vi "LSMcontroller_v59_PIzstage.vi"() -> ()   [LabVIEW 2015] (continued)
                    n3063 = property on="ROI" class="Bool (strict)"("Val(Sgnl)"=FALSE ("x/y scan")) -> ()  [unwired: 2 in, 2 out]
                  }
                }
              }
            }
          }
          event "Xdattype": Value Change {
            n3064 = event-data() -> ()  [unwired: 1 in, 1 out]
            n3065 = case shown="True" "Xdattype" {
              frame False {
              }
              frame True {
                n3066 = stacked-sequence {
                  frame #0 {
                    n3067 = Current VI's Path() -> (path=w6265:path)
                    n3068 = Strip Path(path=w6265) -> (stripped path=w6266:path)  [unwired: 1 out]
                    n3069 = Build Path(base path=w6266, name or relative path="subVIs\\Misc\\Changedataconfig.vi") -> (appended path=w6264:path)
                    n3070 = call <vilib>:"Set Busy.vi"() -> ("error out"=w6262:errorcluster)  [unwired: 10 in, 1 out]
                    n3071 = Open VI Reference(type specifier VI Refnum (for type only)=refnum<vi> refnum, vi path=w6264, error in (no error)=w6262) -> (vi reference=w6257:refnum<vi>, error out=w6259:errorcluster)  [unwired: 3 in]
                    n3072 = call-by-ref "?"(reference=w6257, error in=w6259) -> (reference out=w6261:refnum<vi>, error out=w6260:errorcluster)  [unwired: 12 in]
                    n3073 = Close Reference(reference=w6261, error in (no error)=w6260) -> (error out=w6256:errorcluster)
                    "status" <- w6256
                    n3074 = call <vilib>:"Unset Busy.vi"("error in (no error)"=w6256) -> ()  [unwired: 10 in, 1 out]
                  }
                  frame #1 {
                    n3075 = property on="Xdattype" class="Bool (strict)"("Val(Sgnl)"=FALSE ("x/y scan")) -> ()  [unwired: 2 in, 2 out]
                  }
                }
              }
            }
          }
          event "XautoOD": Value Change {
            n3076 = event-data() -> ()  [unwired: 1 in, 1 out]
            n3077 = case shown="True" "XautoOD" {
              frame False {
              }
              frame True {
                n3078 = stacked-sequence {
                  frame #0 {
                    n3079 = Current VI's Path() -> (path=w6278:path)
                    n3080 = Strip Path(path=w6278) -> (stripped path=w6279:path)  [unwired: 1 out]
                    n3081 = Build Path(base path=w6279, name or relative path="subVIs\\Misc\\ChangeautoODs.vi") -> (appended path=w6277:path)
                    n3082 = call <vilib>:"Set Busy.vi"() -> ("error out"=w6275:errorcluster)  [unwired: 10 in, 1 out]
                    n3083 = Open VI Reference(type specifier VI Refnum (for type only)=refnum<vi> refnum, vi path=w6277, error in (no error)=w6275) -> (vi reference=w6270:refnum<vi>, error out=w6272:errorcluster)  [unwired: 3 in]
                    n3084 = call-by-ref "?"(reference=w6270, error in=w6272) -> (reference out=w6274:refnum<vi>, error out=w6273:errorcluster)  [unwired: 12 in]
                    n3085 = Close Reference(reference=w6274, error in (no error)=w6273) -> (error out=w6269:errorcluster)
                    "status 2" <- w6269
                    n3086 = call <vilib>:"Unset Busy.vi"("error in (no error)"=w6269) -> ()  [unwired: 10 in, 1 out]
                  }
                  frame #1 {
                    n3087 = property on="XautoOD" class="Bool (strict)"("Val(Sgnl)"=FALSE ("x/y scan")) -> ()  [unwired: 2 in, 2 out]
                  }
                }
              }
            }
          }
          event "SetMan": Value Change {
            n3088 = event-data() -> ()  [unwired: 1 in, 1 out]
            n3089 = case shown="True" "SetMan" {
              frame False {
              }
              frame True {
                n3090 = stacked-sequence {
                  frame #0 {
                    w6282 = u16 0 items=["Rectangle", "Circle", "Freeform Boundary", "Freeform Interior"] ("ROI Type")
                    n3091 = local write "ROI Type"(w6282) -> ()
                    n3092 = local read "Square pixels"() -> (w6288:bool)
                    n3093 = case shown="True" w6288 {
                      frame False {
                        n3094 = local read "square matrix"() -> (w6289:bool)
                        n3095 = case shown="False" w6289 {
                          frame False {
                            "ypixels ref" <- "ypixels"
                            "xpixels ref" <- "xpixels"
                          }
                          frame True {
                            n3096 = local read "xpixels"() -> (w6294:i32)
                            n3097 = local read "ypixels"() -> (w6293:i32)
                            n3098 = Max & Min(x=w6294, y=w6293) -> (max(x,y)=w6292:i32)  [unwired: 1 out]
                            n3099 = local write "xpixels ref"(w6292) -> ()
                            n3100 = local write "ypixels ref"(w6292) -> ()
                          }
                        }
                      }
                      frame True {
                        n3101 = local read "square matrix"() -> (w6295:bool)
                        n3102 = case shown="False" w6295 {
                          frame False {
                            n3103 = local read "Vxmax"() -> (w6309:dbl)
                            n3104 = local read "Vx-min"() -> (w6308:dbl)
                            n3105 = local read "Vy-max"() -> (w6304:dbl)
                            n3106 = local read "Vy-min"() -> (w6305:dbl)
                            n3107 = Subtract(x=w6304, y=w6305) -> (x-y=w6306:dbl)
                            n3108 = Subtract(x=w6309, y=w6308) -> (x-y=w6307:dbl)
                            n3109 = Absolute Value(x=w6306) -> (abs(x)=w6297:dbl)
                            n3110 = Absolute Value(x=w6307) -> (abs(x)=w6298:dbl)
                            n3111 = Divide(x=w6298, y=w6297) -> (x/y=w6303:dbl)
                            n3112 = Greater Or Equal?(x=w6298, y=w6297) -> (x >= y?=w6296:bool)
                            n3113 = local read "xpixels"() -> (w6302:i32)
                            n3114 = local read "ypixels"() -> (w6299:i32)
                            n3115 = case shown="False" w6296 {
                              tunnel: w6303 -> [w6314 w6317]
                              tunnel: w6302 -> [w6311 _]
                              tunnel: [w6311 w6316] -> w6301
                              tunnel: [w6310 w6315] -> w6300
                              tunnel: w6299 -> [_ w6315]
                              frame False {
                                n3116 = To Double Precision Float(number=w6311) -> (double precision float=w6313:dbl)
                                n3117 = Divide(x=w6313, y=w6314) -> (x/y=w6312:dbl)
                                n3118 = To Long Integer(number=w6312) -> (32bit integer=w6310:i32)
                              }
                              frame True {
                                n3119 = To Double Precision Float(number=w6315) -> (double precision float=w6319:dbl)
                                n3120 = Multiply(x=w6319, y=w6317) -> (x*y=w6318:dbl)
                                n3121 = To Long Integer(number=w6318) -> (32bit integer=w6316:i32)
                              }
                            }
                            n3122 = local write "ypixels ref"(w6300) -> ()
                            n3123 = local write "xpixels ref"(w6301) -> ()
                          }
                          frame True {
                          }
                        }
                      }
                    }
                    "Vx-max ref" <- "Vxmax"
                    "Vx-min ref" <- "Vx-min"
                    "Vy-max ref" <- "Vy-max"
                    "Vy-min ref" <- "Vy-min"
                    "Angle ref" <- "Angle"
                  }
                  frame #1 {
                    n3124 = property on="SetMan" class="Bool (strict)"("Val(Sgnl)"=FALSE ("Value (Signaling)")) -> ()  [unwired: 2 in, 2 out]
                  }
                }
              }
            }
          }
          event "SetMan 2": Value Change {
            n3125 = event-data() -> ()  [unwired: 1 in, 1 out]
            n3126 = case shown="True" "SetMan 2" {
              frame False {
              }
              frame True {
                n3127 = stacked-sequence {
                  frame #0 {
                    n3128 = local write "Vx-ref"("Vx") -> ()
                    n3129 = local write "Vy-ref"("Vy") -> ()
                  }
                  frame #1 {
                    n3130 = property on="SetMan 2" class="Bool (strict)"("Val(Sgnl)"=FALSE ("Value (Signaling)")) -> ()  [unwired: 2 in, 2 out]
                  }
                }
              }
            }
          }
          event "Reset Coords": Value Change {
            n3131 = event-data() -> ("NewVal"=w6325:bool)  [unwired: 1 in, 5 out]
            n3132 = case shown="True" w6325 {
              frame False {
              }
              frame True {
                n3133 = stacked-sequence {
                  frame #0 {
                    n3134 = local write "xpixels"(256 ("xpixels")) -> ()
                    n3135 = local write "ypixels"(256 ("ypixels")) -> ()
                    n3136 = local write "Vxmax"(9.0 ("Vx-max")) -> ()
                    n3137 = local write "Vx-min"(-9.0 ("Vx-min")) -> ()
                    n3138 = local write "Vy-max"(9.0 ("Vy-max")) -> ()
                    n3139 = local write "Vy-min"(-9.0 ("Vy-min")) -> ()
                    n3140 = local write "Angle"(0.0 ("Angle")) -> ()
                  }
                  frame #1 {
                    n3141 = property on="Reset Coords" class="Bool (strict)"("Value"=FALSE ("TROI")) -> ()  [unwired: 2 in, 2 out]
                  }
                }
              }
            }
          }
          event "TROI": Value Change {
            n3142 = event-data() -> ()  [unwired: 1 in, 1 out]
            n3143 = case shown="True" "TROI" {
              frame False {
              }
              frame True {
                n3144 = stacked-sequence {
                  frame #0 {
                    n3145 = local read "Vy-min ref"() -> (w6339:dbl)
                    n3146 = local read "Vy-max ref"() -> (w6338:dbl)
                    n3147 = local read "Vx-max ref"() -> (w6336:dbl)
                    n3148 = local read "Vx-min ref"() -> (w6337:dbl)
                    n3149 = local read "ypixels ref"() -> (w6341:i32)
                    n3150 = local read "xpixels ref"() -> (w6340:i32)
                    n3151 = local read "Angle ref"() -> (w6335:dbl)
                    n3152 = local write "Angle"(w6335) -> ()
                    n3153 = local write "xpixels"(w6340) -> ()
                    n3154 = local write "Vy-min"(w6339) -> ()
                    n3155 = local write "Vy-max"(w6338) -> ()
                    n3156 = local write "Vx-min"(w6337) -> ()
                    n3157 = local write "ypixels"(w6341) -> ()
                    n3158 = local write "Vxmax"(w6336) -> ()
                  }
                  frame #1 {
                    n3159 = property on="TROI" class="Bool (strict)"("Value"=FALSE ("TROI")) -> ()  [unwired: 2 in, 2 out]
                  }
                }
              }
            }
          }
          event "TROI 2": Value Change {
            n3160 = event-data() -> ()  [unwired: 1 in, 1 out]
            n3161 = case shown="True" "TROI 2" {
              frame False {
              }
              frame True {
                n3162 = stacked-sequence {
                  frame #0 {
                    n3163 = local read "Vx-ref"() -> (w6344:dbl)
                    n3164 = local read "Vy-ref"() -> (w6345:dbl)
                    n3165 = local write "Vx"(w6344) -> ()
                    n3166 = local write "Vy"(w6345) -> ()
                  }
                  frame #1 {
                    n3167 = property on="TROI 2" class="Bool (strict)"("Value"=FALSE ("TROI")) -> ()  [unwired: 2 in, 2 out]
                  }
                }
              }
            }
          }
          event "Square pixels": Value Change {
            n3168 = event-data() -> ()  [unwired: 1 in, 1 out]
            n3169 = case shown="True" "Square pixels" {
              frame False {
              }
              frame True {
                n3170 = property on="square matrix" class="Bool (strict)"("Value"=FALSE ("square matrix")) -> ()  [unwired: 2 in, 2 out]
                n3171 = property on="Square pixels" class="Bool (strict)"("Value"=TRUE ("square matrix")) -> ()  [unwired: 2 in, 2 out]
              }
            }
          }
          event "square matrix": Value Change {
            n3172 = event-data() -> ()  [unwired: 1 in, 1 out]
            n3173 = case shown="True" "square matrix" {
              frame False {
              }
              frame True {
                n3174 = property on="square matrix" class="Bool (strict)"("Value"=TRUE ("square matrix")) -> ()  [unwired: 2 in, 2 out]
                n3175 = property on="Square pixels" class="Bool (strict)"("Value"=FALSE ("square matrix")) -> ()  [unwired: 2 in, 2 out]
              }
            }
          }
          event "up", "downright", "down", "downleft", "right", "left", "upright", "upleft": Value Change {
            n3176 = event-data() -> ()  [unwired: 1 in, 6 out]
            n3177 = local read "downright"() -> (w6358:bool)
            n3178 = local read "downleft"() -> (w6360:bool)
            n3179 = local read "upright"() -> (w6356:bool)
            n3180 = local read "upleft"() -> (w6354:bool)
            n3181 = local read "down"() -> (w6359:bool)
            n3182 = local read "right"() -> (w6357:bool)
            n3183 = local read "left"() -> (w6361:bool)
            n3184 = local read "up"() -> (w6355:bool)
            n3185 = Compound Arithmetic op=OR(w6354, w6355, w6356, w6357, w6358, w6359, w6360, w6361) -> (w6353:bool)
            n3186 = case shown="True" w6353 {
              frame False {
              }
              frame True {
                n3187 = stacked-sequence {
                  frame #0 {
                    n3188 = local read "downright"() -> (w6363:bool)
                    n3189 = local read "downleft"() -> (w6365:bool)
                    n3190 = local read "BigSmall"() -> (w6362:bool)
                    n3191 = local read "upright"() -> (w6367:bool)
                    n3192 = local read "upleft"() -> (w6370:bool)
                    n3193 = local read "down"() -> (w6366:bool)
                    n3194 = local read "right"() -> (w6368:bool)
                    n3195 = local read "left"() -> (w6364:bool)
                    n3196 = local read "up"() -> (w6369:bool)
                    n3197 = call "movestageparams.vi"("command"="get") -> ("Params out"=w6373:T21)  [unwired: 1 in]
                    n3198 = Bundle By Name(cluster=w6373, "upleft"=w6370, "up"=w6369, "upright"=w6367, "right"=w6368, "downright"=w6363, "down"=w6366, "downleft"=w6365, "left"=w6364, "Bigsmall"=w6362) -> (w6374:T21)
                    n3199 = call "movestageparams.vi"("Params in"=w6374, "command"="set") -> ()  [unwired: 1 out]
                  }
                  frame #1 {
                    n3200 = disable-structure shown="Disabled" {
                      frame Disabled {
                        n3201 = call "configuration.vi"("command"="get") -> ("config out"=w6377:T12)  [unwired: 2 in, 1 out]
                        n3202 = in-place {
                          n3203 = in-place-cluster #45(w6377) -> ()  [unwired: 2 out]
                          n3204 = in-place-cluster #45("StageL"="StageL", "StageS"="StageS") -> (w6375:T12)
                        }
                        n3205 = call "configuration.vi"("config in"=w6375, "command"="set") -> ()  [unwired: 1 in, 2 out]
                      }
                      frame Enabled {
                      }
                    }
                  }
                  frame #2 {
                    n3206 = call "movestage.vi"() -> ()  [unwired: 12 in]
                  }
                  frame #3 {
                    w6381 = FALSE ("OK Button")
                    w6382 = FALSE ("OK Button")
                    n3207 = property on="down" class="Bool (strict)"("Value"=w6382) -> ()  [unwired: 2 in, 2 out]
                    n3208 = property on="up" class="Bool (strict)"("Value"=w6382) -> ()  [unwired: 2 in, 2 out]
                    n3209 = property on="right" class="Bool (strict)"("Value"=w6382) -> ()  [unwired: 2 in, 2 out]
                    n3210 = property on="left" class="Bool (strict)"("Value"=w6382) -> ()  [unwired: 2 in, 2 out]
                    n3211 = property on="upright" class="Bool (strict)"("Value"=w6381) -> ()  [unwired: 2 in, 2 out]
                    n3212 = property on="downleft" class="Bool (strict)"("Value"=w6381) -> ()  [unwired: 2 in, 2 out]
                    n3213 = property on="downright" class="Bool (strict)"("Value"=w6381) -> ()  [unwired: 2 in, 2 out]
                    n3214 = property on="upleft" class="Bool (strict)"("Value"=w6381) -> ()  [unwired: 2 in, 2 out]
                  }
                }
              }
            }
          }
          event "finite samples": Value Change {
            n3215 = event-data() -> ("NewVal"=w6383:bool)  [unwired: 1 in]
            n3216 = flat-sequence {
              tunnel: w6383 -> [w6384]
              frame #0 {
                n3217 = case shown="True" w6384 {
                  frame False {
                    w6385 = FALSE ("wavdet")
                    n3218 = property on="continuous" class="Bool (strict)"("Value"=TRUE ("continuous for display")) -> ()  [unwired: 2 in, 2 out]
                    n3219 = property on="wavdet" class="Bool (strict)"("Value"=w6385) -> ()  [unwired: 2 in, 2 out]
                    n3220 = property on="save\ndata" class="Bool (strict)"("Value"=w6385) -> ()  [unwired: 2 in, 2 out]
                    n3221 = property on="# of frames" class="DigNum (strict)"("DisabledEnum"=T7."Disabled and Grayed Out" ("Disabled")) -> ()  [unwired: 2 in, 2 out]
                    n3222 = property on="save\ndata" class="Bool (strict)"("DisabledEnum"=T7."Disabled and Grayed Out" ("Disabled")) -> ()  [unwired: 2 in, 2 out]
                    "Save tab" <- enum32{"withsave", "withoutsave"}."withsave" ("Save tab")
                  }
                  frame True {
                    w6392 = FALSE ("continuous for display")
                    n3223 = property on="continuous" class="Bool (strict)"("Value"=w6392) -> ()  [unwired: 2 in, 2 out]
                    n3224 = property on="wavdet" class="Bool (strict)"("Value"=w6392) -> ()  [unwired: 2 in, 2 out]
                    n3225 = local write "Save tab"(enum32{"withsave", "withoutsave"}."withsave" ("Save tab")) -> ()
                    n3226 = property on="save\ndata" class="Bool (strict)"("DisabledEnum"=T7."Enabled" ("Disabled")) -> ()  [unwired: 2 in, 2 out]
                    n3227 = property on="save\ndata" class="Bool (strict)"("Value"=TRUE ("save\ndata")) -> ()  [unwired: 2 in, 2 out]
                    n3228 = property on="# of frames" class="DigNum (strict)"("DisabledEnum"=T7."Enabled" ("Disabled")) -> ()  [unwired: 2 in, 2 out]
                  }
                }
              }
              frame #1 {
                n3229 = local read "finite samples"() -> (w6401:bool)
                n3230 = local read "continuous"() -> (w6400:bool)
                n3231 = local read "wavdet"() -> (w6399:bool)
                n3232 = call "2pparameters.vi"("command"="get") -> ("params out"=w6395:T11)  [unwired: 1 in]
                n3233 = Bundle By Name(cluster=w6395, "finite"=w6401, "cont"=w6400, "wavdet"=w6399) -> (w6398:T11)
                n3234 = call "2pparameters.vi"("Params in"=w6398, "command"="set") -> ()  [unwired: 1 out]
              }
            }
          }
          event "continuous": Value Change {
            n3235 = event-data() -> ("NewVal"=w6402:bool)  [unwired: 1 in]
            n3236 = flat-sequence {
              tunnel: w6402 -> [w6403]
              frame #0 {
                n3237 = case shown="True" w6403 {
                  frame False {
                    n3238 = property on="finite samples" class="Bool (strict)"("Value"=TRUE ("finite samples for recording")) -> ()  [unwired: 2 in, 2 out]
                    n3239 = property on="save\ndata" class="Bool (strict)"("Value"=TRUE ("save\ndata")) -> ()  [unwired: 2 in, 2 out]
                    n3240 = property on="wavdet" class="Bool (strict)"("Value"=FALSE ("wavdet")) -> ()  [unwired: 2 in, 2 out]
                    n3241 = local write "Save tab"(enum32{"withsave", "withoutsave"}."withsave" ("Save tab")) -> ()
                    n3242 = property on="# of frames" class="DigNum (strict)"("DisabledEnum"=T7."Enabled" ("Disabled")) -> ()  [unwired: 2 in, 2 out]
                    n3243 = property on="save\ndata" class="Bool (strict)"("DisabledEnum"=T7."Enabled" ("Disabled")) -> ()  [unwired: 2 in, 2 out]
                  }
                  frame True {
                    w6410 = FALSE ("finite samples for recording")
                    n3244 = property on="finite samples" class="Bool (strict)"("Value"=w6410) -> ()  [unwired: 2 in, 2 out]
                    n3245 = property on="wavdet" class="Bool (strict)"("Value"=w6410) -> ()  [unwired: 2 in, 2 out]
                    n3246 = property on="save\ndata" class="Bool (strict)"("Value"=w6410) -> ()  [unwired: 2 in, 2 out]
                    n3247 = local write "Save tab"(enum32{"withsave", "withoutsave"}."withsave" ("Save tab")) -> ()
                    n3248 = property on="# of frames" class="DigNum (strict)"("DisabledEnum"=T7."Disabled and Grayed Out" ("Disabled")) -> ()  [unwired: 2 in, 2 out]
                    n3249 = property on="save\ndata" class="Bool (strict)"("DisabledEnum"=T7."Disabled and Grayed Out" ("Disabled")) -> ()  [unwired: 2 in, 2 out]
                  }
                }
              }
              frame #1 {
                n3250 = local read "finite samples"() -> (w6420:bool)
                n3251 = local read "continuous"() -> (w6419:bool)
                n3252 = local read "wavdet"() -> (w6418:bool)
                n3253 = call "2pparameters.vi"("command"="get") -> ("params out"=w6414:T11)  [unwired: 1 in]
                n3254 = Bundle By Name(cluster=w6414, "finite"=w6420, "cont"=w6419, "wavdet"=w6418) -> (w6417:T11)
                n3255 = call "2pparameters.vi"("Params in"=w6417, "command"="set") -> ()  [unwired: 1 out]
              }
            }
          }
          event "wavdet": Value Change {
            n3256 = event-data() -> ("NewVal"=w6421:bool)  [unwired: 1 in]
            n3257 = flat-sequence {
              tunnel: w6421 -> [w6422]
              frame #0 {
                n3258 = case shown="False" w6422 {
                  frame False {
                    n3259 = property on="finite samples" class="Bool (strict)"("Value"=TRUE ("finite samples for recording")) -> ()  [unwired: 2 in, 2 out]
                    n3260 = property on="continuous" class="Bool (strict)"("Value"=FALSE ("continuous")) -> ()  [unwired: 2 in, 2 out]
                    n3261 = local write "Save tab"(enum32{"withsave", "withoutsave"}."withsave" ("Save tab")) -> ()
                    n3262 = property on="save\ndata" class="Bool (strict)"("DisabledEnum"=T7."Enabled" ("Disabled")) -> ()  [unwired: 2 in, 2 out]
                    n3263 = property on="# of frames" class="DigNum (strict)"("DisabledEnum"=T7."Enabled" ("Disabled")) -> ()  [unwired: 2 in, 2 out]
                    n3264 = property on="save\ndata" class="Bool (strict)"("Value"=TRUE ("save\ndata")) -> ()  [unwired: 2 in, 2 out]
                  }
                  frame True {
                    w6431 = FALSE ("finite samples for recording")
                    n3265 = property on="finite samples" class="Bool (strict)"("Value"=w6431) -> ()  [unwired: 2 in, 2 out]
                    n3266 = property on="continuous" class="Bool (strict)"("Value"=w6431) -> ()  [unwired: 2 in, 2 out]
                    n3267 = property on="save\ndata" class="Bool (strict)"("DisabledEnum"=T7."Enabled" ("Disabled")) -> ()  [unwired: 2 in, 2 out]
                    n3268 = local write "Save tab"(enum32{"withsave", "withoutsave"}."withsave" ("Save tab")) -> ()
                    n3269 = property on="# of frames" class="DigNum (strict)"("DisabledEnum"=T7."Disabled" ("Disabled")) -> ()  [unwired: 2 in, 2 out]
                    n3270 = property on="save\ndata" class="Bool (strict)"("Value"=TRUE ("save\ndata")) -> ()  [unwired: 2 in, 2 out]
                  }
                }
              }
              frame #1 {
                n3271 = local read "finite samples"() -> (w6434:bool)
                n3272 = local read "continuous"() -> (w6435:bool)
                n3273 = local read "wavdet"() -> (w6436:bool)
                n3274 = call "2pparameters.vi"("command"="get") -> ("params out"=w6440:T11)  [unwired: 1 in]
                n3275 = Bundle By Name(cluster=w6440, "finite"=w6434, "cont"=w6435, "wavdet"=w6436) -> (w6437:T11)
                n3276 = call "2pparameters.vi"("Params in"=w6437, "command"="set") -> ()  [unwired: 1 out]
              }
            }
          }
          event "cursors": Value Change {
            n3277 = event-data() -> ()  [unwired: 1 in, 5 out]
            n3278 = case shown="True" "cursors" {
              frame False {
                n3279 = property on="img_CH1" class="IntGraph (strict)"("Active Cursor"=u32 0, "Cursor.Cursor Style"=u8 0 ("Cursor Style"), "Cursor.Cursor Point Style"=u8 0 ("Cursor Point Style")) -> ("Cursor.Cursor Position:Cursor X"=w6445:dbl, "Cursor.Cursor Position:Cursor Y"=w6446:dbl)  [unwired: 2 in, 2 out]
                n3280 = property on="img_CH2" class="IntGraph (strict)"("Active Cursor"=u32 0, "Cursor.Cursor Style"=u8 0 ("Cursor Style"), "Cursor.Cursor Point Style"=u8 0 ("Cursor Point Style")) -> ()  [unwired: 2 in, 2 out]
                n3281 = local write "cursor x [pixel]"(w6445) -> ()
                n3282 = local write "cursor y [pixel]"(w6446) -> ()
              }
              frame True {
                n3283 = stacked-sequence {
                  frame #0 {
                    n3284 = call "2pparameters.vi"("command"="get") -> ("params out"=w6461:T11)  [unwired: 1 in]
                    n3285 = Unbundle By Name(w6461) -> ("Xpixels Img"=w6462:i32, "Ypixels Img"=w6459:i32)
                    n3286 = To Double Precision Float(number=w6459) -> (double precision float=w6453:dbl)
                    n3287 = To Double Precision Float(number=w6462) -> (double precision float=w6458:dbl)
                    n3288 = Divide(x=w6453, y=2.0) -> (x/y=w6454:dbl)
                    n3289 = Divide(x=w6458, y=2.0) -> (x/y=w6456:dbl)
                    n3290 = Round To Nearest(number=w6454) -> (nearest integer value=w6452:dbl)
                    n3291 = Round To Nearest(number=w6456) -> (nearest integer value=w6455:dbl)
                    n3292 = property on="img_CH1" class="IntGraph (strict)"("Active Cursor"=u32 0, "Cursor.Cursor Style"=u8 8 ("Cursor Style"), "Cursor.Cursor Point Style"=u8 5 ("Cursor Point Style"), "Cursor.Cursor Position:Cursor X"=w6455, "Cursor.Cursor Position:Cursor Y"=w6452, "Cursor.Visible"=TRUE) -> ()  [unwired: 2 in, 2 out]
                  }
                  frame #1 {
                    n3293 = call "2pparameters.vi"("command"="get") -> ("params out"=w6481:T11)  [unwired: 1 in]
                    n3294 = call "2pparameters.vi"("command"="get") -> ("params out"=w6479:T11)  [unwired: 1 in]
                    n3295 = property on="img_CH1" class="IntGraph (strict)"("Active Cursor"=u32 0, "Cursor.Cursor Style"=u8 8 ("Cursor Style"), "Cursor.Cursor Point Style"=u8 5 ("Cursor Point Style")) -> ("Cursor.Cursor Position:Cursor X"=w6474:dbl, "Cursor.Cursor Position:Cursor Y"=w6473:dbl, "Cursor.Cursor Index"=w6496:i32, "Cursor.Cursor Plot"=w6495:i32, "Cursor.Visible"=w6466:bool)  [unwired: 2 in, 2 out]
                    "cursor x [pixel]" <- w6474
                    "cursor y [pixel]" <- w6473
                    n3296 = Unbundle By Name(w6481) -> ("Vy-max Img"=w6483:dbl, "Vy-min Img"=w6470:dbl, "Ypixels Img"=w6485:i32)
                    n3297 = Unbundle By Name(w6479) -> ("VX-max Img"=w6480:dbl, "Vx-min Img"=w6468:dbl, "Xpixels Img"=w6484:i32)
                    n3298 = Subtract(x=w6483, y=w6470) -> (x-y=w6488:dbl)
                    n3299 = Subtract(x=w6480, y=w6468) -> (x-y=w6486:dbl)
                    n3300 = local read "img_CH2"() -> (w6492:sgl[][])
                    n3301 = To Double Precision Float(number=w6484) -> (double precision float=w6487:dbl)
                    n3302 = local read "img_CH1"() -> (w6493:sgl[][])
                    n3303 = To Double Precision Float(number=w6485) -> (double precision float=w6489:dbl)
                    n3304 = Index Array(array=w6493, index (row)=w6496, index (col)=w6495) -> (element=→"value CH 1":sgl)
                    n3305 = Index Array(array=w6492, index (row)=w6496, index (col)=w6495) -> (element=→"value CH 2":sgl)
                    n3306 = Divide(x=w6486, y=w6487) -> (x/y=w6490:dbl)
                    n3307 = Divide(x=w6488, y=w6489) -> (x/y=w6491:dbl)
                    n3308 = Multiply(x=w6474, y=w6490) -> (x*y=w6469:dbl)
                    n3309 = Multiply(x=w6473, y=w6491) -> (x*y=w6472:dbl)
                    n3310 = property on="img_CH2" class="IntGraph (strict)"("Active Cursor"=u32 0, "Cursor.Cursor Style"=u8 8 ("Cursor Style"), "Cursor.Cursor Point Style"=u8 5 ("Cursor Point Style"), "Cursor.Cursor Position:Cursor X"=w6474, "Cursor.Cursor Position:Cursor Y"=w6473, "Cursor.Visible"=w6466) -> ()  [unwired: 2 in, 2 out]
                    n3311 = Add(x=w6469, y=w6468) -> (x+y=w6467:dbl)
                    n3312 = Add(x=w6472, y=w6470) -> (x+y=w6471:dbl)
                    n3313 = local write "Vx-ref"(w6467) -> ()
                    n3314 = local write "Vy-ref"(w6471) -> ()
                  }
                }
              }
            }
          }
          event "img_CH1": Cursor Move {
            n3315 = event-data() -> ("CursIdx"=w6501:i32)  [unwired: 1 in]
            n3316 = Equal To 0?(x=w6501) -> (x = 0?=w6502:bool)
            n3317 = case shown="True" w6502 {
              frame False {
              }
              frame True {
                n3318 = call "2pparameters.vi"("command"="get") -> ("params out"=w6522:T11)  [unwired: 1 in]
                n3319 = call "2pparameters.vi"("command"="get") -> ("params out"=w6524:T11)  [unwired: 1 in]
                n3320 = property on="img_CH1" class="IntGraph (strict)"("Active Cursor"=u32 0, "Cursor.Cursor Style"=u8 8 ("Cursor Style"), "Cursor.Cursor Point Style"=u8 5 ("Cursor Point Style")) -> ("Cursor.Cursor Position:Cursor X"=w6511:dbl, "Cursor.Cursor Position:Cursor Y"=w6510:dbl, "Cursor.Cursor Plot"=w6530:i32, "Cursor.Cursor Index"=w6529:i32, "Cursor.Visible"=w6503:bool)  [unwired: 2 in, 2 out]
                n3321 = Unbundle By Name(w6522) -> ("Vy-max Img"=w6520:dbl, "Vy-min Img"=w6509:dbl, "Ypixels Img"=w6518:i32)
                n3322 = Unbundle By Name(w6524) -> ("VX-max Img"=w6523:dbl, "Vx-min Img"=w6504:dbl, "Xpixels Img"=w6519:i32)
                n3323 = Subtract(x=w6520, y=w6509) -> (x-y=w6515:dbl)
                n3324 = Subtract(x=w6523, y=w6504) -> (x-y=w6517:dbl)
                n3325 = local write "cursor x [pixel]"(w6511) -> ()
                n3326 = local write "cursor y [pixel]"(w6510) -> ()
                n3327 = To Double Precision Float(number=w6519) -> (double precision float=w6516:dbl)
                n3328 = To Double Precision Float(number=w6518) -> (double precision float=w6514:dbl)
                n3329 = local read "img_CH2"() -> (w6531:sgl[][])
                n3330 = local read "img_CH1"() -> (w6534:sgl[][])
                n3331 = Index Array(array=w6531, index (row)=w6530, index (col)=w6529) -> (element=w6532:sgl)
                n3332 = Index Array(array=w6534, index (row)=w6530, index (col)=w6529) -> (element=w6533:sgl)
                n3333 = Divide(x=w6517, y=w6516) -> (x/y=w6513:dbl)
                n3334 = Divide(x=w6515, y=w6514) -> (x/y=w6512:dbl)
                n3335 = local write "value CH 2"(w6532) -> ()
                n3336 = Multiply(x=w6511, y=w6513) -> (x*y=w6506:dbl)
                n3337 = local write "value CH 1"(w6533) -> ()
                n3338 = Multiply(x=w6510, y=w6512) -> (x*y=w6508:dbl)
                n3339 = Add(x=w6506, y=w6504) -> (x+y=w6505:dbl)
                n3340 = local write "Vx-ref"(w6505) -> ()
                n3341 = Add(x=w6508, y=w6509) -> (x+y=w6507:dbl)
                n3342 = property on="img_CH2" class="IntGraph (strict)"("Active Cursor"=u32 0, "Cursor.Cursor Style"=u8 8 ("Cursor Style"), "Cursor.Cursor Point Style"=u8 5 ("Cursor Point Style"), "Cursor.Cursor Position:Cursor X"=w6511, "Cursor.Cursor Position:Cursor Y"=w6510, "Cursor.Visible"=w6503) -> ()  [unwired: 2 in, 2 out]
                n3343 = local write "Vy-ref"(w6507) -> ()
              }
            }
          }
          event "img_CH2": Cursor Move {
            n3344 = event-data() -> ("CursIdx"=w6538:i32)  [unwired: 1 in]
            n3345 = Equal To 0?(x=w6538) -> (x = 0?=w6539:bool)
            n3346 = case shown="True" w6539 {
              frame False {
              }
              frame True {
                n3347 = property on="img_CH2" class="IntGraph (strict)"("Active Cursor"=u32 0, "Cursor.Cursor Style"=u8 8 ("Cursor Style"), "Cursor.Cursor Point Style"=u8 5 ("Cursor Point Style")) -> ("Cursor.Cursor Position:Cursor X"=w6547:dbl, "Cursor.Cursor Position:Cursor Y"=w6548:dbl, "Cursor.Cursor Plot"=w6567:i32, "Cursor.Cursor Index"=w6566:i32, "Cursor.Visible"=w6540:bool)  [unwired: 2 in, 2 out]
                n3348 = call "2pparameters.vi"("command"="get") -> ("params out"=w6559:T11)  [unwired: 1 in]
                n3349 = call "2pparameters.vi"("command"="get") -> ("params out"=w6561:T11)  [unwired: 1 in]
                n3350 = local read "img_CH1"() -> (w6571:sgl[][])
                n3351 = local read "img_CH2"() -> (w6568:sgl[][])
                n3352 = local write "cursor x [pixel]"(w6547) -> ()
                n3353 = local write "cursor y [pixel]"(w6548) -> ()
                n3354 = Unbundle By Name(w6559) -> ("Vy-max Img"=w6557:dbl, "Vy-min Img"=w6542:dbl, "Ypixels Img"=w6555:i32)
                n3355 = Unbundle By Name(w6561) -> ("VX-max Img"=w6560:dbl, "Vx-min Img"=w6545:dbl, "Xpixels Img"=w6556:i32)
                n3356 = Index Array(array=w6571, index (row)=w6567, index (col)=w6566) -> (element=w6570:sgl)
                n3357 = Index Array(array=w6568, index (row)=w6567, index (col)=w6566) -> (element=w6569:sgl)
                n3358 = local write "value CH 2"(w6569) -> ()
                n3359 = local write "value CH 1"(w6570) -> ()
                n3360 = Subtract(x=w6557, y=w6542) -> (x-y=w6552:dbl)
                n3361 = Subtract(x=w6560, y=w6545) -> (x-y=w6554:dbl)
                n3362 = To Double Precision Float(number=w6556) -> (double precision float=w6553:dbl)
                n3363 = To Double Precision Float(number=w6555) -> (double precision float=w6551:dbl)
                n3364 = Divide(x=w6554, y=w6553) -> (x/y=w6550:dbl)
                n3365 = Divide(x=w6552, y=w6551) -> (x/y=w6549:dbl)
                n3366 = Multiply(x=w6547, y=w6550) -> (x*y=w6546:dbl)
                n3367 = Multiply(x=w6548, y=w6549) -> (x*y=w6543:dbl)
                n3368 = property on="img_CH1" class="IntGraph (strict)"("Active Cursor"=u32 0, "Cursor.Cursor Style"=u8 8 ("Cursor Style"), "Cursor.Cursor Point Style"=u8 5 ("Cursor Point Style"), "Cursor.Cursor Position:Cursor X"=w6547, "Cursor.Cursor Position:Cursor Y"=w6548, "Cursor.Visible"=w6540) -> ()  [unwired: 2 in, 2 out]
                n3369 = Add(x=w6546, y=w6545) -> (x+y=→"Vx-ref":dbl)
                n3370 = Add(x=w6543, y=w6542) -> (x+y=→"Vy-ref":dbl)
              }
            }
          }
          event "auto shutter": Value Change {
            n3371 = event-data() -> ()  [unwired: 1 in, 6 out]
            n3372 = call "2pparameters.vi"("command"="get") -> ("params out"=w6577:T11)  [unwired: 1 in]
            n3373 = in-place {
              n3374 = in-place-cluster #46(w6577) -> ()  [unwired: 1 out]
              n3375 = local read "auto shutter"() -> (w6579:bool)
              n3376 = in-place-cluster #46("autoshutter"=w6579) -> (w6575:T11)
            }
            n3377 = call "2pparameters.vi"("Params in"=w6575, "command"="set") -> ()  [unwired: 1 out]
          }
          event "auto OD": Value Change {
            n3378 = event-data() -> ()  [unwired: 1 in, 6 out]
            n3379 = call "2pparameters.vi"("command"="get") -> ("params out"=w6582:T11)  [unwired: 1 in]
            n3380 = in-place {
              n3381 = in-place-cluster #47(w6582) -> ()  [unwired: 1 out]
              n3382 = local read "auto OD"() -> (w6584:bool)
              n3383 = in-place-cluster #47("auto OD"=w6584) -> (w6580:T11)
            }
            n3384 = call "2pparameters.vi"("Params in"=w6580, "command"="set") -> ()  [unwired: 1 out]
          }
          event "ODfilt": Value Change {
            n3385 = event-data() -> ("OldVal"=w6585:u16)  [unwired: 1 in, 5 out]
            n3386 = local read "ODfilt"() -> (w6586:u16)
            n3387 = call "2pparameters.vi"("command"="get") -> ("params out"=w6589:T11)  [unwired: 1 in]
            n3388 = call "filterwheelcontrol_nothorlabslib.vi"("Current OD filt"=w6585, "New ODfilt"=w6586) -> ()  [unwired: 1 in]
            n3389 = in-place {
              in-place-border: w6586 -> [w6591]
              n3390 = in-place-cluster #48(w6589) -> ()  [unwired: 1 out]
              n3391 = in-place-cluster #48("ODfilt"=w6591) -> (w6587:T11)
            }
            n3392 = call "2pparameters.vi"("Params in"=w6587, "command"="set") -> ()  [unwired: 1 out]
          }
          event "Exit": Value Change {
            n3393 = event-data() -> ()  [unwired: 1 in, 5 out]
          }
        }
        n3394 = Wait (ms)(milliseconds to wait=u32 50) -> ()  [unwired: 1 out]
      }
      n3395 = while {
        stop <- w69 stop-if-true
        # "Waveform generation"
        n3396 = event shown="[2] \"AO channels\": Value Change" {
          selector: _ -> [_ _ _ _ _ _ _ _ _ _ _ _ _ _ _ _ _]
          dyn-events: _ -> [_ _ _ _ _ _ _ _ _ _ _ _ _ _ _ _ _]
          timeout: _ -> [_ _ _ _ _ _ _ _ _ _ _ _ _ _ _ _ _]
          tunnel: [_ _ _ _ _ _ _ _ _ _ _ _ _ _ _ _ w2042] -> w69
          event Timeout {
            n3397 = event-data() -> ()  [unwired: 1 in, 3 out]
          }
          event "Add AO wave": Value Change {
            n3398 = event-data() -> ("NewVal"=w70:bool)  [unwired: 1 in, 5 out]
            n3399 = case shown="True" w70 {
              frame False {
              }
              frame True {
                n3400 = stacked-sequence {
                  frame #0 {
                    n3401 = local read "Measurement"() -> (w71:T4)
                    n3402 = case shown="\"Lifetime (contour)\"" w71 {
                      frame "X-Y-t movie", Default {
                        n3403 = local read "avpp"() -> (w92:i32)
                        n3404 = local read "Angle ref"() -> (w91:dbl)
                        n3405 = local read "ROI Type"() -> (w90:u16)
                        n3406 = local read "xpixels ref"() -> (w87:i32)
                        n3407 = local read "Vx-min ref"() -> (w86:dbl)
                        n3408 = local read "Vx-max ref"() -> (w85:dbl)
                        n3409 = local read "ypixels ref"() -> (w83:i32)
                        n3410 = local read "Vy-min ref"() -> (w84:dbl)
                        n3411 = local read "Vy-max ref"() -> (w80:dbl)
                        n3412 = local read "Sampling rate"() -> (w74:dbl)
                        n3413 = local read "finite samples"() -> (w75:bool)
                        n3414 = local read "continuous"() -> (w78:bool)
                        n3415 = local read "wavdet"() -> (w79:bool)
                        n3416 = local read "# of frames"() -> (w77:i32)
                        n3417 = local read "maxbufferAI"() -> (w76:i32)
                        n3418 = local read "Override AI buffer"() -> (w72:bool)
                        n3419 = call "2pparameters.vi"("command"="get") -> ("params out"=w89:T11)  [unwired: 1 in]
                        n3420 = Bundle By Name(cluster=w89, "type"="X-Y-t movie", "avpp"=w92, "Angle Img"=w91, "Xpixels Img"=w87, "Vx-min Img"=w86, "VX-max Img"=w85, "Ypixels Img"=w83, "Vy-min Img"=w84, "Vy-max Img"=w80, "srate"=w74, "srate Img"=w74, "finite"=w75, "cont"=w78, "wavdet"=w79, "measpoints"=w77, "maxbufferAI"=w76, "Drawing Mode"=w90, "Vz-reset"=0.0, "AIoverride"=w72) -> (w81:T11)
                        n3421 = call "2pparameters.vi"("Params in"=w81, "command"="set") -> ()  [unwired: 1 out]
                      }
                      frame "X-Y-Z stack" {
                        n3422 = call "2pparameters.vi"("command"="get") -> ("params out"=w96:T11)  [unwired: 1 in]
                        n3423 = Bundle By Name(cluster=w96, "type"="X-Y-Z stack") -> (w94:T11)
                        n3424 = call "2pparameters.vi"("Params in"=w94, "command"="set") -> ()  [unwired: 1 out]
                      }
                      frame "Lifetime (scan)" {
                        n3425 = call "2pparameters.vi"("command"="get") -> ("params out"=w101:T11)  [unwired: 1 in]
                        n3426 = Bundle By Name(cluster=w101, "type"="Lifetime (scan)") -> (w99:T11)
                        n3427 = call "2pparameters.vi"("Params in"=w99, "command"="set") -> ()  [unwired: 1 out]
                      }
                      frame "Lifetime (contour)" {
                        n3428 = local read "Vy-min draw"() -> (w111:dbl)
                        n3429 = local read "Vy-max draw"() -> (w110:dbl)
                        n3430 = local read "Vx-min draw"() -> (w113:dbl)
                        n3431 = local read "Vx-max draw"() -> (w112:dbl)
                        n3432 = local read "xpixels ref"() -> (w109:i32)
                        n3433 = local read "ypixels ref"() -> (w108:i32)
                        n3434 = local read "ROI Type"() -> (w107:u16)
                        n3435 = local read "srateAODOtt"() -> (w118:dbl)
                        n3436 = local read "# of frames"() -> (w123:i32)
                        n3437 = local read "refreshtime"() -> (w115:dbl)
                        n3438 = local read "Pel"() -> (w106:dbl)
                        n3439 = local read "bin"() -> (w121:dbl)
                        n3440 = local read "Override AI buffer"() -> (w104:bool)
                        n3441 = local read "finite samples"() -> (w130:bool)
                        n3442 = local read "srateAODOtt"() -> (w117:dbl)
                        n3443 = local read "srateAODOtt"() -> (w124:dbl)
                        n3444 = local read "continuous"() -> (w129:bool)
                        n3445 = local read "Angle ref"() -> (w114:dbl)
                        n3446 = local read "wavdet"() -> (w131:bool)
                        n3447 = local read "Vx-ref"() -> (w126:dbl)
                        n3448 = local read "Vy-ref"() -> (w128:dbl)
                        n3449 = local read "avpp"() -> (w127:i32)
                        n3450 = call "tt_timeandsamples.vi"("bin"=w121, "refreshtime"=w115, "srateAODOtt"=w118, "tot#ofsamples"=w123) -> ("refreshrate"=w119:dbl, "refreshbuffer"=w120:i32, "timetracecycles"=w125:i32)  [unwired: 5 in]
                        n3451 = local read "bin"() -> (w122:dbl)
                        n3452 = call "2pparameters.vi"("command"="get") -> ("params out"=w134:T11)  [unwired: 1 in]
                        n3453 = Bundle By Name(cluster=w134, "Drawing Mode"=w107, "measpoints"=w123, "tt_cycles"=w125, "refreshbuffer"=w120, "refreshrate"=w119, "Vx-ref"=w126, "Vy-ref"=w128, "srate"=w117, "finite"=w130, "cont"=w129, "wavdet"=w131, "avpp"=w127, "srateAODO"=w124, "bufferAI"=w120, "bin"=w122, "Angle Img"=w114, "Vxminref"=w113, "Vxmaxref"=w112, "Vyminref"=w111, "Vymaxref"=w110, "Xpixels Img"=w109, "Ypixels Img"=w108, "Pel"=w106, "Vz-reset"=0.0, "AIoverride"=w104, "type"="Lifetime (contour)") -> (w132:T11)
                        n3454 = Reciprocal(x=w119) -> (1/x=w116:dbl)
                        n3455 = local write "refreshtime"(w116) -> ()
                        n3456 = call "2pparameters.vi"("Params in"=w132, "command"="set") -> ()  [unwired: 1 out]
                      }
                      frame "X-Y-Z-t movie" {
                      }
                      frame "linescan" {
                      }
                      frame "Timetrace" {
                        n3457 = local read "Vy-min draw"() -> (w144:dbl)
                        n3458 = local read "Vy-max draw"() -> (w143:dbl)
                        n3459 = local read "Vx-min draw"() -> (w146:dbl)
                        n3460 = local read "Vx-max draw"() -> (w145:dbl)
                        n3461 = local read "xpixels ref"() -> (w142:i32)
                        n3462 = local read "ypixels ref"() -> (w141:i32)
                        n3463 = local read "ROI Type"() -> (w140:u16)
                        n3464 = local read "srateAODOtt"() -> (w151:dbl)
                        n3465 = local read "# of frames"() -> (w156:i32)
                        n3466 = local read "refreshtime"() -> (w148:dbl)
                        n3467 = local read "Pel"() -> (w139:dbl)
                        n3468 = local read "bin"() -> (w154:dbl)
                        n3469 = local read "Override AI buffer"() -> (w137:bool)
                        n3470 = local read "finite samples"() -> (w163:bool)
                        n3471 = local read "srateAODOtt"() -> (w150:dbl)
                        n3472 = local read "srateAODOtt"() -> (w157:dbl)
                        n3473 = local read "continuous"() -> (w162:bool)
                        n3474 = local read "Angle ref"() -> (w147:dbl)
                        n3475 = local read "wavdet"() -> (w164:bool)
                        n3476 = local read "Vx-ref"() -> (w159:dbl)
                        n3477 = local read "Vy-ref"() -> (w161:dbl)
                        n3478 = local read "avpp"() -> (w160:i32)
                        n3479 = call "tt_timeandsamples.vi"("bin"=w154, "refreshtime"=w148, "srateAODOtt"=w151, "tot#ofsamples"=w156) -> ("refreshrate"=w152:dbl, "refreshbuffer"=w153:i32, "timetracecycles"=w158:i32)  [unwired: 5 in]
                        n3480 = local read "bin"() -> (w155:dbl)
                        n3481 = call "2pparameters.vi"("command"="get") -> ("params out"=w167:T11)  [unwired: 1 in]
                        n3482 = Bundle By Name(cluster=w167, "Drawing Mode"=w140, "measpoints"=w156, "tt_cycles"=w158, "refreshbuffer"=w153, "refreshrate"=w152, "Vx-ref"=w159, "Vy-ref"=w161, "srate"=w150, "finite"=w163, "cont"=w162, "wavdet"=w164, "avpp"=w160, "srateAODO"=w157, "bufferAI"=w153, "bin"=w155, "Angle Img"=w147, "Vxminref"=w146, "Vxmaxref"=w145, "Vyminref"=w144, "Vymaxref"=w143, "Xpixels Img"=w142, "Ypixels Img"=w141, "Pel"=w139, "Vz-reset"=0.0, "AIoverride"=w137, "type"="Timetrace") -> (w165:T11)
                        n3483 = Reciprocal(x=w152) -> (1/x=w149:dbl)
                        n3484 = local write "refreshtime"(w149) -> ()
                        n3485 = call "2pparameters.vi"("Params in"=w165, "command"="set") -> ()  [unwired: 1 out]
                      }
                      frame "Lifetime (point)" {
                      }
                    }
                  }
                  frame #1 {
                    w170 = FALSE ("wavdet")
                    n3486 = call "2pparameters.vi"("command"="get") -> ("params out"=w174:T11)  [unwired: 1 in]
                    n3487 = Bundle By Name(cluster=w174, "finite"=w170, "cont"=w170, "wavdet"=TRUE) -> (w171:T11)
                    n3488 = call "2pparameters.vi"("Params in"=w171, "command"="set") -> ()  [unwired: 1 out]
                  }
                  frame #2 {
                    # "change active waveform numbers array"
                    n3489 = local read "AO channels"() -> (w181:u32)
                    n3490 = call "2pparameters.vi"("command"="get") -> ("params out"=w179:T11)  [unwired: 1 in]
                    n3491 = in-place {
                      in-place-border: w181 -> [w185]
                      in-place-border: [w182] -> w176
                      n3492 = in-place-cluster #49(w179) -> ("aAO"=w184:u32[])
                      n3493 = call "add channel to active arrayv2.vi"("line array in"=w184, "line to add"=w185) -> ("line array out"=w183:u32[], "addition"=w182:bool)  [unwired: 1 out]
                      n3494 = in-place-cluster #49("aAO"=w183) -> (w177:T11)
                    }
                    n3495 = local write "addAO"(w176) -> ()
                    n3496 = call "2pparameters.vi"("Params in"=w177, "command"="set") -> ()  [unwired: 1 out]
                  }
                  frame #3 {
                    # "update GUI"
                    n3497 = local read "addAO"() -> (w186:bool)
                    n3498 = case shown="True" w186 {
                      frame False {
                      }
                      frame True {
                        n3499 = call "Used AO lines.vi"() -> ("used AO names"=w190:string[], "used AO lines"=w192:tag[])  [unwired: 2 in]
                        n3500 = control-ref of="Analog Lines Plot"() -> (w191:refnum<vi>)
                        n3501 = control-ref of="Digital Lines Plot"() -> (w189:refnum<vi>)
                        n3502 = call "Used DO lines.vi"() -> ("used DO names"=w188:string[], "used DO lines"=w187:tag[])  [unwired: 2 in]
                        n3503 = local write "Analog Used Lines"(w192) -> ()
                        n3504 = local write "Analog Used Names"(w190) -> ()
                        n3505 = local write "Digital Used Lines"(w187) -> ()
                        n3506 = local write "Digital Used Names"(w188) -> ()
                        n3507 = call "prepDOWaveplot.vi"("DigitalGraph in"=w189, "used DO names"=w188) -> ()  [unwired: 1 in]
                        n3508 = call "prepAOWaveplot.vi"("WaveformGraph in"=w191, "Analog Used Names"=w190) -> ()  [unwired: 1 in]
                      }
                    }
                  }
                  frame #4 {
                    n3509 = local read "addAO"() -> (w193:bool)
                    n3510 = case shown="True" w193 {
                      frame False {
                      }
                      frame True {
                        # "add parameters\nto parameter array"
                        n3511 = local read "Build analog waveform tabs"() -> (w194:enum32{"Square", "Triangle", "Matlab"})
                        n3512 = case shown="\"Square\", Default" w194 {
                          frame "Square", Default {
                            w207 = 0.0 ("Offset (V)")
                            n3513 = local read "Meastab"() -> (w196:enum32{"X-Y Image", "Linescan", "Timetrace"})
                            n3514 = call "waveformparamsv2.vi"("command"="get") -> ("Params out"=w205:T15)  [unwired: 4 in, 2 out]
                            n3515 = Unbundle By Name(w205) -> ("AO parameters"=w202:T16)
                            n3516 = case shown="\"Timetrace\"" w196 {
                              tunnel: [w218 w219] -> w195
                              frame "X-Y Image", Default {
                                n3517 = local read "Sampling rate"() -> (w218:dbl)
                              }
                              frame "Timetrace" {
                                n3518 = local read "srateAODOtt"() -> (w219:dbl)
                              }
                            }
                            n3519 = local read "Start amplitude (V)"() -> (w215:dbl)
                            n3520 = local read "phase shift (ms)"() -> (w208:dbl)
                            n3521 = local read "Step size (V)"() -> (w213:dbl)
                            n3522 = local read "Baseline (V)"() -> (w214:dbl)
                            n3523 = local read "Period (ms)"() -> (w211:dbl)
                            n3524 = local read "padding value"() -> (w198:dbl)
                            n3525 = local read "Repeats"() -> (w217:dbl)
                            n3526 = local read "DC (%)"() -> (w212:dbl)
                            n3527 = local read "Cycles"() -> (w216:dbl)
                            n3528 = local read "Pulses"() -> (w209:dbl)
                            n3529 = Index Array(array=w202, index=0) -> (element=w203:T17)
                            n3530 = Bundle By Name(cluster=w203, "AOtab"=0.0 ("Repeats"), "Repeats"=w217, "Cycles"=w216, "Start amplitude (V)"=w215, "Baseline (V)"=w214, "Step size (V)"=w213, "DC (%)"=w212, "Sampling frequency (Hz)"=w195, "Period (ms)"=w211, "Offset (V)"=w207, "Amplitude (V)"=w207, "Frequency"=w207, "Tri Repeats"=w207, "phase shift (ms)"=w208, "Pulses"=w209, "Matlab wave file"=path "", "padding value"=w198) -> (w200:T17)
                            n3531 = Build Array(w200) -> (w199:T16)
                            n3532 = call "waveformparamsv2.vi"("command"="add AO", "add AO"=w199) -> ()  [unwired: 3 in, 3 out]
                          }
                          frame "Matlab" {
                            w225 = 0.0 ("Repeats")
                            n3533 = local read "Meastab"() -> (w221:enum32{"X-Y Image", "Linescan", "Timetrace"})
                            n3534 = call "waveformparamsv2.vi"("command"="get") -> ("Params out"=w232:T15)  [unwired: 4 in, 2 out]
                            n3535 = Unbundle By Name(w232) -> ("AO parameters"=w229:T16)
                            n3536 = case shown="\"Timetrace\"" w221 {
                              tunnel: [w235 w236] -> w220
                              frame "X-Y Image", Default {
                                n3537 = local read "Sampling rate"() -> (w235:dbl)
                              }
                              frame "Timetrace" {
                                n3538 = local read "srateAODOtt"() -> (w236:dbl)
                              }
                            }
                            n3539 = local read "Matlab waveform path"() -> (w222:path)
                            n3540 = local read "Matlab padding value"() -> (w224:dbl)
                            n3541 = Index Array(array=w229, index=0) -> (element=w230:T17)
                            n3542 = call "matlabwfexistsdialogue.vi"("Matlab waveform path"=w222) -> ("mtalab waveform path out"=w223:path)
                            n3543 = Bundle By Name(cluster=w230, "AOtab"=2.0 ("Repeats"), "Repeats"=w225, "Cycles"=w225, "Start amplitude (V)"=w225, "Baseline (V)"=w225, "Step size (V)"=w225, "DC (%)"=w225, "Sampling frequency (Hz)"=w220, "Period (ms)"=w225, "Offset (V)"=w225, "Amplitude (V)"=w225, "Frequency"=w225, "Tri Repeats"=w225, "phase shift (ms)"=w225, "Pulses"=w225, "Matlab wave file"=w223, "padding value"=w224) -> (w227:T17)
                            n3544 = Build Array(w227) -> (w226:T16)
                            n3545 = call "waveformparamsv2.vi"("command"="add AO", "add AO"=w226) -> ()  [unwired: 3 in, 3 out]
                          }
                          frame "Triangle" {
                            w242 = 0.0 ("Offset (V)")
                            n3546 = local read "Meastab"() -> (w238:enum32{"X-Y Image", "Linescan", "Timetrace"})
                            n3547 = call "waveformparamsv2.vi"("command"="get") -> ("Params out"=w254:T15)  [unwired: 4 in, 2 out]
                            n3548 = Unbundle By Name(w254) -> ("AO parameters"=w251:T16)
                            n3549 = case shown="\"Timetrace\"" w238 {
                              tunnel: [w256 w257] -> w237
                              frame "X-Y Image", Default {
                                n3550 = local read "Sampling rate"() -> (w256:dbl)
                              }
                              frame "Timetrace" {
                                n3551 = local read "srateAODOtt"() -> (w257:dbl)
                              }
                            }
                            n3552 = local read "Tri padding value"() -> (w240:dbl)
                            n3553 = local read "Amplitude (V)"() -> (w245:dbl)
                            n3554 = local read "Tri Phase (s)"() -> (w241:dbl)
                            n3555 = local read "Tri Repeats"() -> (w243:dbl)
                            n3556 = local read "Frequency"() -> (w244:dbl)
                            n3557 = local read "Offset (V)"() -> (w246:dbl)
                            n3558 = Index Array(array=w251, index=0) -> (element=w252:T17)
                            n3559 = Bundle By Name(cluster=w252, "AOtab"=1.0 ("Repeats"), "Repeats"=w242, "Cycles"=w242, "Start amplitude (V)"=w242, "Baseline (V)"=w242, "Step size (V)"=w242, "DC (%)"=w242, "Sampling frequency (Hz)"=w237, "Period (ms)"=w242, "Offset (V)"=w246, "Amplitude (V)"=w245, "Frequency"=w244, "Tri Repeats"=w243, "phase shift (ms)"=w242, "Pulses"=w242, "Matlab wave file"=path "", "Tri phase"=w241, "padding value"=w240) -> (w249:T17)
                            n3560 = Build Array(w249) -> (w248:T16)
                            n3561 = call "waveformparamsv2.vi"("command"="add AO", "add AO"=w248) -> ()  [unwired: 3 in, 3 out]
                          }
                        }
                      }
                    }
                  }
                  frame #5 {
                    n3562 = local read "addAO"() -> (w258:bool)
                    n3563 = case shown="True" w258 {
                      frame False {
                      }
                      frame True {
                        # "add waveform to waveform array; correct waveform lengths and plot"
                        n3564 = local read "Meastab"() -> (w262:enum32{"X-Y Image", "Linescan", "Timetrace"})
                        n3565 = local read "Build analog waveform tabs"() -> (w272:enum32{"Square", "Triangle", "Matlab"})
                        n3566 = case shown="\"Timetrace\"" w262 {
                          tunnel: [w280 w281] -> w261
                          frame "X-Y Image", Default {
                            n3567 = local read "Sampling rate"() -> (w280:dbl)
                          }
                          frame "Timetrace" {
                            n3568 = local read "srateAODOtt"() -> (w281:dbl)
                          }
                        }
                        n3569 = call "waveformparamsv2.vi"("command"="get last AO") -> ("last AO"=w274:T17)  [unwired: 4 in, 2 out]
                        n3570 = case shown="\"Matlab\"" w272 {
                          tunnel: w274 -> [w284 w286 w288]
                          tunnel: [w283 w285 w287] -> w273
                          frame "Square", Default {
                            n3571 = call "generateRampedSquareWave_fromAOparameters.vi"("AO params"=w284) -> ("Waveform"=w283:waveform(dbl))  [unwired: 1 out]
                          }
                          frame "Triangle" {
                            n3572 = call "generateTriWave_fromAOparameters.vi"("AO params"=w286) -> ("Waveform"=w285:waveform(dbl))  [unwired: 1 out]
                          }
                          frame "Matlab" {
                            n3573 = call "matlabAOwffromparam.vi"("Cluster"=w288) -> ("Waveform"=w287:waveform(dbl))  [unwired: 1 out]
                          }
                        }
                        n3574 = property on="refwf" class="Ring (strict)"() -> ("RingText.Text"=w265:string)  [unwired: 2 in, 2 out]
                        n3575 = call "waveformsAObuffer.vi"("command"="get") -> ("AO wf out"=w278:waveform(dbl)[])  [unwired: 1 in]
                        n3576 = Build Array (concatenate)(w278, w273) -> (w275:waveform(dbl)[])
                        n3577 = call "waveformsDObuffer.vi"("command"="get") -> ("DO wf out"=w270:digitalwaveform[])  [unwired: 1 in]
                        n3578 = call "correctwaveformsizetemp.vi"("new sampling frequency (Hz)"=w261, "start"=FALSE, "reference waveforms to"=w265, "Analog waveforms in"=w275, "stop"=FALSE, "Digital waveforms in"=w270) -> ("analog wf out"=w268:waveform(dbl)[], "Digital wf out"=w266:digitalwaveform[], "measpoints"=w263:i32)
                        n3579 = local write "Analog Lines Plot"(w268) -> ()
                        n3580 = call "GetNumCamFramesv2.vi"("Digital Waveform Graph"=w266) -> ("Numeric"=w267:i32)  [unwired: 10 in]
                        n3581 = local write "Digital Lines Plot"(w266) -> ()
                        n3582 = call "waveformsAObuffer.vi"("AO wf in"=w268, "command"="set") -> ()  [unwired: 1 out]
                        n3583 = call "waveformsDObuffer.vi"("DO wf in"=w266, "command"="set") -> ()  [unwired: 1 out]
                        n3584 = local write "Total Camera Frames"(w267) -> ()
                        n3585 = local read "wavdet"() -> (w264:bool)
                        n3586 = case shown="True" w264 {
                          tunnel: w263 -> [_ w282]
                          frame False {
                          }
                          frame True {
                            n3587 = local write "# of frames"(w282) -> ()
                          }
                        }
                      }
                    }
                  }
                  frame #6 {
                    w289 = FALSE ("addAO")
                    # "set signaling boolean to false"
                    n3588 = local read "finite samples"() -> (w290:bool)
                    n3589 = local read "continuous"() -> (w291:bool)
                    n3590 = local read "wavdet"() -> (w292:bool)
                    n3591 = call "2pparameters.vi"("command"="get") -> ("params out"=w295:T11)  [unwired: 1 in]
                    n3592 = Bundle By Name(cluster=w295, "finite"=w290, "cont"=w291, "wavdet"=w292) -> (w293:T11)
                    n3593 = local write "addAO"(w289) -> ()
                    n3594 = property on="Add AO wave" class="Bool (strict)"("Val(Sgnl)"=w289) -> ()  [unwired: 2 in, 2 out]
                    n3595 = call "2pparameters.vi"("Params in"=w293, "command"="set") -> ()  [unwired: 1 out]
                  }
                }
              }
            }
          }
          event "AO channels": Value Change {
            n3596 = event-data() -> ()  [unwired: 1 in, 6 out]
            n3597 = local read "AO channels"() -> (w297:u32)
            n3598 = call "2pparameters.vi"("command"="get") -> ("params out"=w299:T11)  [unwired: 1 in]
            n3599 = Unbundle By Name(w299) -> ("aAO"=w298:u32[])
            n3600 = Search 1D Array(1D array=w298, element=w297) -> (index of element=w301:i32)  [unwired: 1 in]
            n3601 = Equal?(x=w301, y=-1.0) -> (x = y?=w302:bool)
            n3602 = case shown="False" w302 {
              tunnel: w301 -> [w304 _]
              frame False {
                n3603 = call "waveformparamsv2.vi"("command"="get") -> ("Params out"=w311:T15)  [unwired: 4 in, 2 out]
                n3604 = Unbundle By Name(w311) -> ("AO parameters"=w310:T16)
                n3605 = Index Array(array=w310, index=w304) -> (element=w327:T17)
